vi "Configuration Utility.vi"() -> ()   [LabVIEW 2013, in "RT Temperature Controller.lvlib"]
doc: "This is the main VI for the configuration editor."
uses:
  RT Temperature Controller.lvlib
  Controls/StateCluster.ctl
  <vilib>/NI/Tag Bus Data Framework/Configuration Editor/Classes/SystemConfigRepo/SystemConfigRepo.lvclass
  <vilib>/CEF_TreeControl/Node/NodeRef.ctl
  <vilib>/CEF_TreeControl/Node/NISE_CEF_Node.lvclass
  <vilib>/CEF_TreeControl/Node/UserEventRef.ctl
  <vilib>/CEF_TreeControl/Controls/EventCluster.ctl
  subVI/SplashScreen/splash screen.ctl
  subVI/SplashScreen/notifier data.ctl
  Controls/add message.ctl
  Controls/MoveMessage.ctl
  <vilib>/NI/Tag Bus Module Framework/plugin discovery singleton/class discovery singleton methods.ctl
  <vilib>/NI/Tag Bus Data Framework/Configuration Editor/Classes/Systems/Systems.lvclass
  <vilib>/NI/Tag Bus Data Framework/Framework Configuration Classes/platypus configuration/systems cluster.ctl
  <vilib>/NI/Tag Bus Data Framework/Framework Configuration Classes/system configuration/PL_System Configuration.lvclass
  <vilib>/NI/Tag Bus Data Framework/Framework Configuration Classes/platypus configuration/targets cluster.ctl
  <vilib>/NI/Tag Bus Data Framework/Framework Configuration Classes/target configuration/PL_Target Configuration.lvclass
  <vilib>/NI/Tag Bus Data Framework/Framework Configuration Classes/platypus configuration/engines cluster.ctl
  <vilib>/NI/Module Execution Interface/Engine Configuration/engine configuration.lvclass
  <vilib>/NI/Tag Bus Module Framework/module configuration/TBM module configuration.lvclass
  <vilib>/NI/Tag Bus Data Framework/Configuration Editor/Classes/SystemConfigRepo/SystemConfigRepo.lvclass/SystemConfigRepo.ctl
  <vilib>/CEF_TreeControl/Repository/NISE_CEF_Repository.lvclass
  <vilib>/NI/AMC/Create Single Message.vi
  <vilib>/NI/AMC/Update Message Routing Info.vi
  <vilib>/NI/AMC/Read Termination Message.vi
  <vilib>/NI/Tag Bus Data Framework/Configuration Editor/subVIs/Glyphs Status.ctl
  <vilib>/NI/Tag Bus Data Framework/Configuration Editor/subVIs/Add status to name.vi
  <vilib>/NI/AMC/Send Message.vi
  <vilib>/NI/AMC/Globals.vi
  <vilib>/NI/Tag Bus Data Framework/Configuration Editor/Classes/Module editor node/module editor node.lvclass
  <vilib>/NI/Tag Bus Data Framework/Configuration Editor/Classes/EngineTags/EngineTags.lvclass
  <vilib>/NI/Module Timing Source/timing source/TBM timing source.lvclass
  <vilib>/NI/Tag Bus Data Framework/Configuration Editor/Classes/TBM Configuration Node/TBM Configuration Node.lvclass
  <vilib>/NI/Tag Bus Module Framework/root configuration/TBM configuration.lvclass
  <vilib>/NI/Tag Bus Data Framework/Configuration Editor/Classes/Targets/Targets.lvclass
  <vilib>/NI/Tag Bus Data Framework/Configuration Editor/Classes/Engine Parent/Engine Parent Editor Node.lvclass
  <vilib>/NI/Tag Bus Module Framework/channel/TBM channel.lvclass
  <vilib>/NI/AMC/AMC.lvlib
  <vilib>/CEF_TreeControl/NISE_CEF_TreeControl.lvlib
  subVI/SplashScreen/splash screen.lvlib
  <vilib>/NI/Tag Bus Data Framework/Framework Configuration Classes/class cache/PL_class cache.lvlib
  <vilib>/NI/Tag Bus Module Framework/plugin discovery singleton/class discovery singleton.lvlib
  <vilib>/NI/Tag Bus Data Framework/Configuration Editor/PL Framework Configuration Tool.lvlib
  <vilib>/NI/Tag Bus Data Framework/Framework Configuration Classes/platypus configuration/PLConfigurationSerializer.lvlib
panel:
  in  "Exit":bool
  in  "View":string(tree)
  # "Tag Bus Configuration Editor"
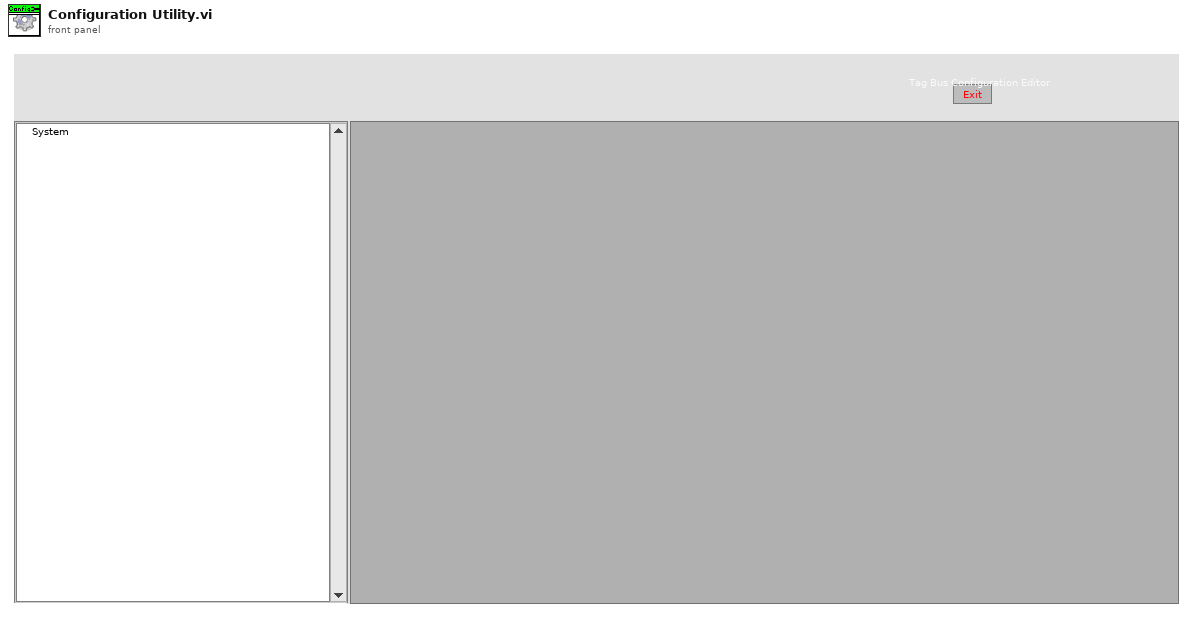
[diagram p1: front panel]
types:
  T1 = enum32{"Invalid", "Standard", "Closed", "Hidden", "Minimized", "Maximized"}
  T2 = typedef "RT Temperature Controller.lvlib/StateCluster.ctl" = cluster{"repository":refnum<class "SystemConfigRepo.lvclass">, "root":T3, "unsaved changes":bool, "current path":path, "user event ref":T4, "glyph path":path[], "SplashScreen":T5, "classes cache":path}
  T3 = typedef "NISE_CEF_Node.lvclass/NodeRef.ctl" = refnum<data-value>
  T4 = typedef "NISE_CEF_Node.lvclass/UserEventRef.ctl" = refnum<user-event>
  T5 = typedef "RT Temperature Controller.lvlib/splash screen.lvlib/splash screen.ctl" = cluster{"reference":refnum<vi>, "update notifier":refnum<notifier>, "Initialized":bool}
  T6 = typedef "AMC.lvlib/Message Queue.ctl" = refnum<queue>
  T7 = typedef "RT Temperature Controller.lvlib/splash screen.lvlib/notifier data.ctl" = cluster{"Text":string, "percent":dbl}
  T8 = typedef "NISE_CEF_TreeControl.lvlib/EventCluster.ctl" = cluster{"command":string, "data":string}
  T9 = typedef "class discovery singleton.lvlib/class discovery singleton methods.ctl" = enum16{"add search paths", "load class by name", "list available classes", "get class path"}
  T10 = typedef "PLConfigurationSerializer.lvlib/systems cluster.ctl" = cluster{"System Configuration":refnum<class "PL_System Configuration.lvclass">, "targets":T11[]}
  T11 = typedef "PLConfigurationSerializer.lvlib/targets cluster.ctl" = cluster{"Target Configuration":refnum<class "PL_Target Configuration.lvclass">, "engines":T12[]}
  T12 = typedef "PLConfigurationSerializer.lvlib/engines cluster.ctl" = cluster{"engine configuration":refnum<class "engine configuration.lvclass">, "modules":refnum<class "TBM module configuration.lvclass">[]}
  T13 = cluster{"node id":string, "RightClickPath":string}
  T14 = typedef "RT Temperature Controller.lvlib/add message.ctl" = cluster{"node type":string, "to add to":string}
  T15 = typedef "RT Temperature Controller.lvlib/MoveMessage.ctl" = cluster{"node ref":T3, "new parent":T3}
  T16 = typedef "RT Temperature Controller.lvlib/FilePaths.ctl" = cluster{"glyphs":path[], "classes":path, "classes cache":path}
  T17 = typedef "PL_class cache.lvlib/cache definition.ctl" = cluster{"configuration":T18, "class cache data":T19}
  T18 = typedef "PL_class cache.lvlib/cache search configuration.ctl" = cluster{"Search Paths":path[], "Folders to Exclude":string[], "full class list":path[]}
  T19 = typedef "PL_class cache.lvlib/cached class information.ctl" = cluster{"targets":T20[], "engines":T21[], "modules":T21[], "ignored class list":path[]}
  T20 = typedef "PL_class cache.lvlib/target class metadata.ctl" = cluster{"file name":string, "fully qualified name":string, "menu display name":string, "configuration class name":string}
  T21 = typedef "PL_class cache.lvlib/class metadata.ctl" = cluster{"file name":string, "fully qualified name":string, "menu display name":string, "configuration class":string, "instances allowed":i32, "supported targets":T22[]}
  T22 = typedef "TBM configuration.lvclass/Target Types.ctl" = enum16{"Windows", "Mac", "Linux", "Linux RT ARM", "VxWorks", "Pharlap", "Other", "Linux RT x64"}
  T23 = typedef "NISE_CEF_Node.lvclass/Summary.ctl" = cluster{"ID":string, "parent ID":string, "node type":string, "text":string, "additional text":string, "glyph":string, "depth":i32}
  T24 = typedef "LVPoint32TypeDef.ctl" = cluster{"Horizontal":i32, "Vertical":i32}
  T25 = cluster{"data name":string, "drag data":variant}[]
  T26 = typedef "NISE_CEF_Node.lvclass/NodeMenuOptions.ctl" = cluster{"removable":bool, "movable":bool, "duplicate":bool}
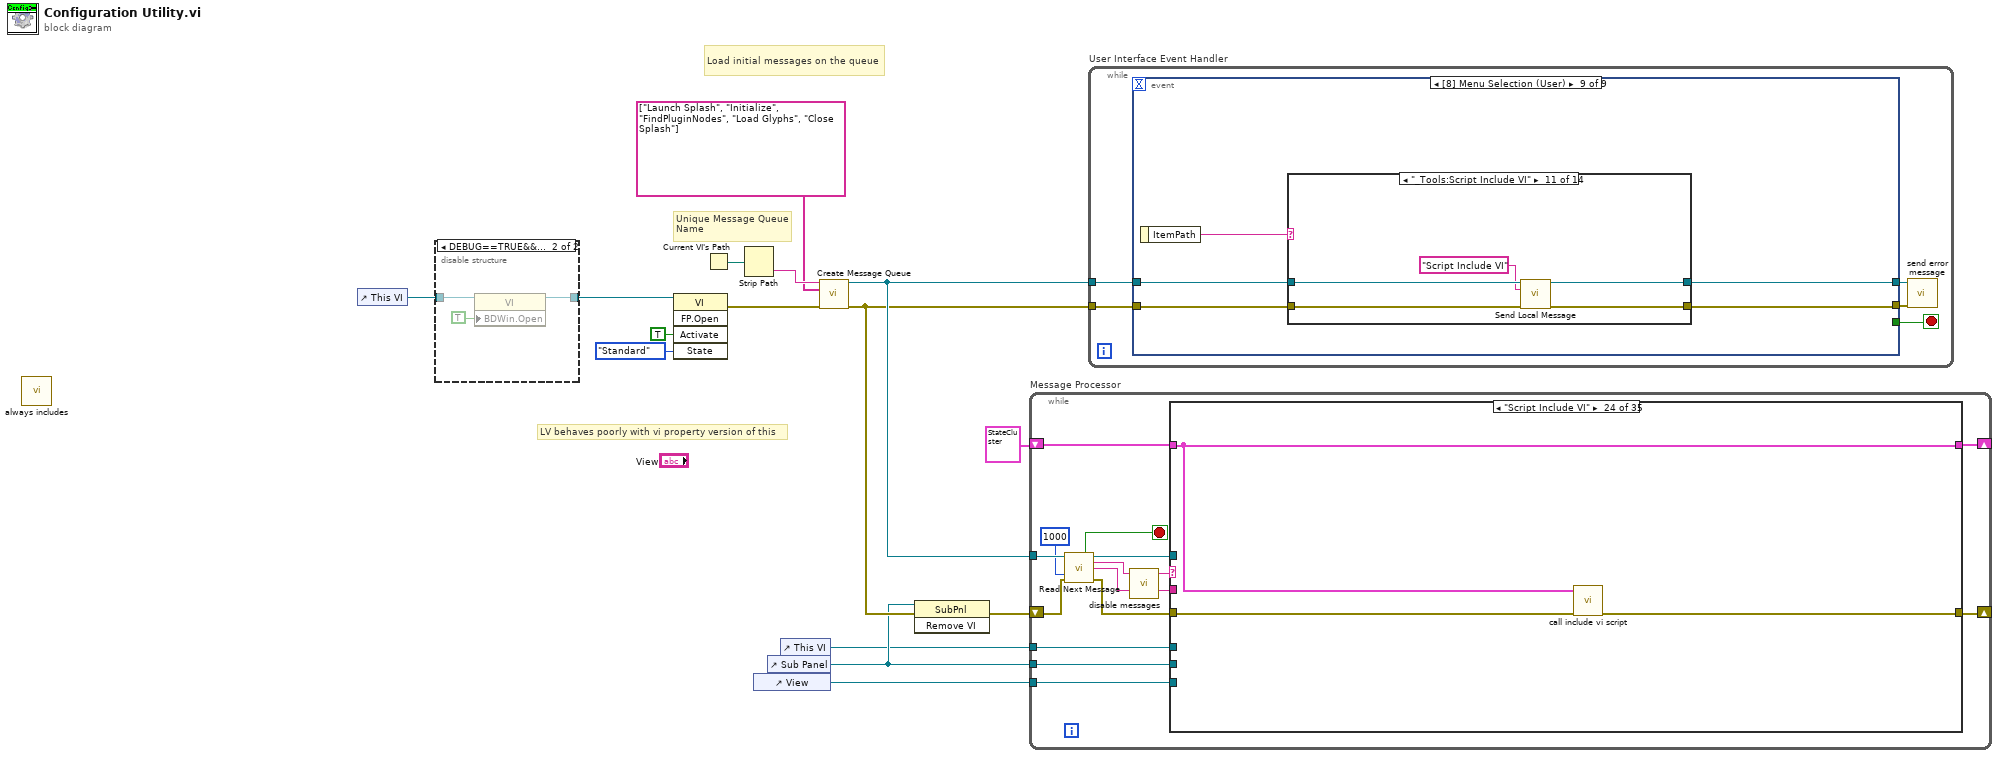
[diagram p0: block diagram]
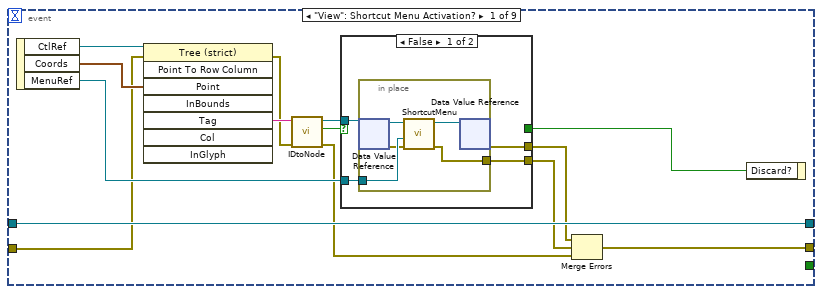
[diagram p3: hidden frame]
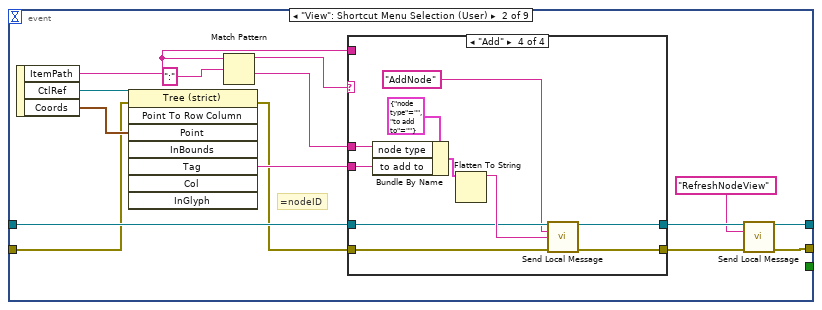
[diagram p5: hidden frame]
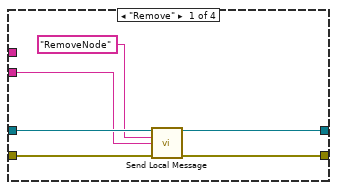
[diagram p6: hidden frame]
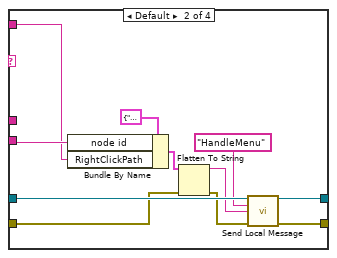
[diagram p7: hidden frame]
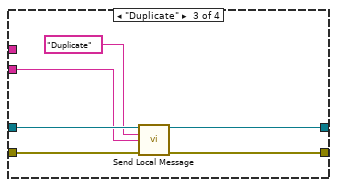
[diagram p8: hidden frame]
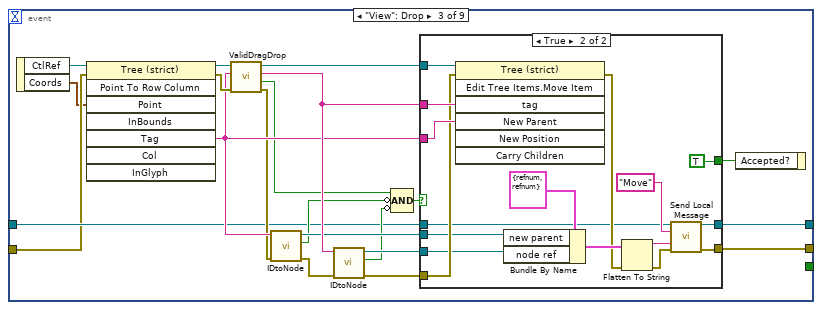
[diagram p9: hidden frame]
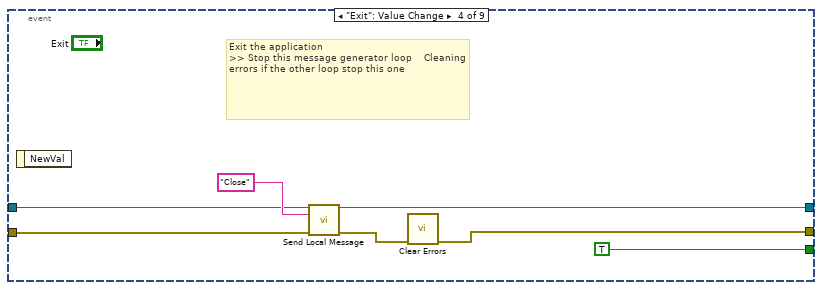
[diagram p11: hidden frame]
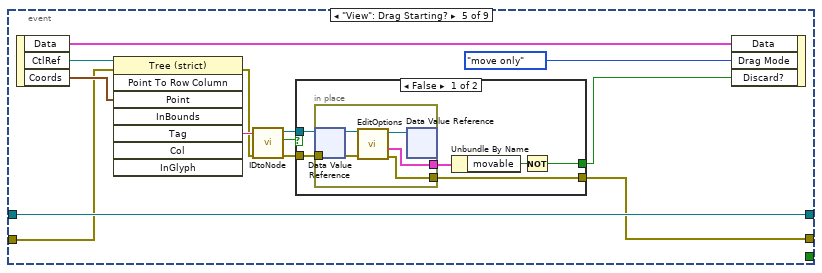
[diagram p12: hidden frame]
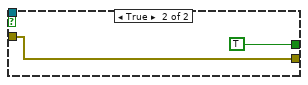
[diagram p13: hidden frame]
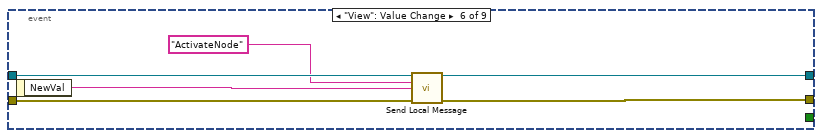
[diagram p14: hidden frame]
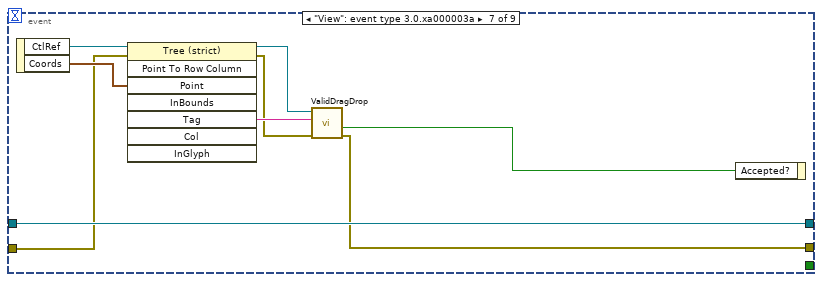
[diagram p15: hidden frame]
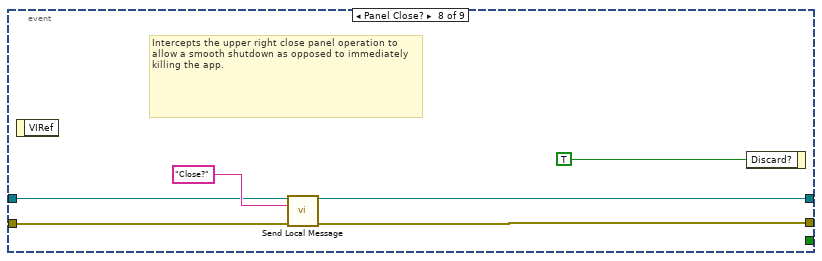
[diagram p16: hidden frame]
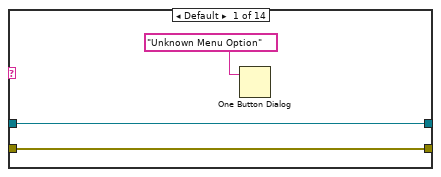
[diagram p17: hidden frame]
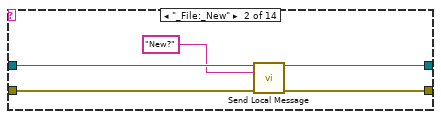
[diagram p18: hidden frame]
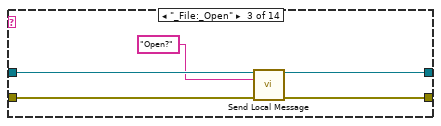
[diagram p19: hidden frame]
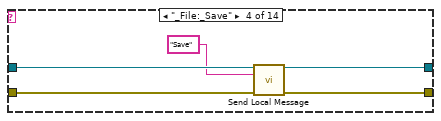
[diagram p20: hidden frame]
diagram:
  # "LV behaves poorly with vi property version of this"
  # "Unique Message Queue Name"
  # "Load initial messages on the queue"
  n1 = call "always includes.vi"() -> ()  [unwired: 12 in]
  n2 = control-ref of="This VI"() -> (w5:refnum<vi>)
  n3 = disable-structure shown="DEBUG==TRUE&&RUN_TIME_ENGINE==False" {
    disable-tunnel: [w16 w19] -> w6
    disable-tunnel: w5 -> [w16 w18]
    frame condition #0 (active) {
    }
    frame condition #1 {
      n4 = property class="VI"(reference=w18, "BDWin.Open"=TRUE ("Block Diagram Window:Open")) -> (reference out=w19:refnum<vi>)  [unwired: 1 in, 1 out]
    }
  }
  n5 = invoke class="VI" method="FP.Open"(reference=w6, "Activate"=TRUE ("Activate?"), "State"=T1."Standard") -> (error out=w9:errorcluster)  [unwired: 2 in, 4 out]
  n6 = Current VI's Path() -> (path=w14:path)
  n7 = Strip Path(path=w14) -> (name=w15:string)  [unwired: 1 out]
  n8 = control-ref of="View"() -> (w4:refnum<vi>)
  n9 = control-ref of="Sub Panel"() -> (w2:refnum<vi>)
  n10 = control-ref of="This VI"() -> (w1:refnum<vi>)
  n11 = call <vilib>:"Create Message Queue.vi"("message queue name"=w15, "initial message names"=string[] ["Launch Splash", "Initialize", "FindPluginNodes", "Load Glyphs", "Close Splash"], "error in"=w9) -> ("message queue out"=w12:T6, "error out"=w10:errorcluster)  [unwired: 11 in]
  n12 = invoke class="SubPnl" method="Remove VI"(reference=w2, error in=w10) -> (error out=w3:errorcluster)  [unwired: 1 in, 2 out]
  n13 = while "Message Processor" {
    shift-right: [w32] -> _
    shift-left: w3 -> [w31]
    tunnel: w12 -> [w30]
    shift-right: [w28] -> _
    shift-left: T2 {"repository"=refnum, "root"=refnum, "unsaved changes"=FALSE, "current path"=path "", "user event ref"=refnum, "glyph path"=[], "SplashScreen"={"reference"=refnum, "update notifier"=refnum, "Initialized"=FALSE}, "classes cache"=path ""} -> [w27]
    tunnel: w1 -> [w22]
    tunnel: w2 -> [w21]
    tunnel: w4 -> [w20]
    stop <- w34 stop-if-true
    n14 = call <vilib>:"Read Next Message.vi"("message queue in"=w30, "timeout (1 ms)"=1000, "error in"=w31) -> ("exit process?"=w34:bool, "message queue out"=w26:T6, "message name"=w23:string, "message value"=w25:string, "error out"=w33:errorcluster)  [unwired: 5 in, 3 out]
    n15 = call "disable messages.vi"("message to check"=w23) -> ("message out"=w24:string)  [unwired: 10 in]
    n16 = case shown="\"Script Include VI\"" w24 {
      selector: w24 -> [_ w38 _ _ _ _ _ _ _ _ _ w156 _ _ _ w278 _ _ _ _ _ _ _ _ _ _ _ _ _ _ _ _ _ _ _]
      tunnel: w25 -> [_ _ _ _ _ _ _ _ w112 _ _ _ _ _ _ _ _ w321 _ _ w383 _ w420 _ _ w461 w473 w491 _ w516 _ _ w563 w586 _]
      tunnel: w33 -> [w36 w41 w43 w50 w69 w76 w97 w103 w113 w139 w143 w153 w190 w202 w237 w270 w297 w326 w343 w348 w381 w395 w422 w437 w440 w459 w472 w492 w504 w515 w541 w551 w562 w585 w591]
      tunnel: [w36 w41 w43 w53 w54 w83 w98 w106 errorcluster {"status"=FALSE, "code"=0, "source"=""} ("error out") w137 w143 w158 w193 w195 w230 w281 w308 w325 w342 w350 w368 w394 w413 w436 w440 w460 w474 w495 w504 w514 w537 w548 w561 w584 w590] -> w32
      tunnel: [w35 w37 w42 w51 w56 w79 w88 w104 w114 w136 w142 w154 w191 w194 w229 w282 w309 w322 w344 w349 w384 w391 w421 w438 w439 w442 w475 w493 w505 w508 w546 w550 w559 w587 w589] -> w28
      tunnel: w27 -> [w35 w37 w42 w52 w70 w79 w89 w104 w114 w136 w142 w155 w189 w203 w238 w277 w304 w323 w344 w349 w384 w392 w421 w438 w439 w458 w475 w494 w506 w508 w546 w550 w559 w587 w589]
      tunnel: w26 -> [_ _ _ _ _ _ w99 w105 w116 w138 _ w157 w192 w201 w236 w267 w307 w324 _ w351 _ w393 w409 _ _ _ _ _ _ _ _ _ w560 w583 _]
      tunnel: w22 -> [_ _ _ w44 w62 _ w86 _ _ _ _ _ _ _ _ _ _ _ _ _ _ _ _ _ _ _ _ _ _ _ w536 _ _ _ _]
      tunnel: w21 -> [_ _ _ _ _ _ _ _ w107 w129 _ w145 _ _ _ w268 w295 _ _ _ _ _ _ _ _ _ _ _ _ w509 _ w547 w552 _ _]
      tunnel: w20 -> [_ _ _ _ _ w82 _ _ _ _ _ w144 _ _ _ _ _ _ _ _ _ _ w408 _ _ w443 w468 w486 _ w510 w540 _ _ _ _]
      frame "", "Idle" {
      }
      frame "Missing Message Handler", Default {
        # "Call this case if a message is received that is not handled by any other case. Typically this is a programming error as a result of a typo or unhandled message/missing message handler."
        n17 = Format Into String(format string="Internal Error: Missing message handler for '%s\" message." ("message"), w38) -> (resulting string=w40:string)  [unwired: 2 in, 1 out]
        n18 = One Button Dialog(message=w40) -> ()  [unwired: 2 out]
      }
      frame "------------Generic Operations------------" {
        # "Dummy case to add a seperation in the Case Structure menu"
      }
      frame "Launch Splash" {
        n19 = invoke class="VI" method="FP.Center"(reference=w44, error in=w50) -> (reference out=w48:refnum<vi>, error out=w47:errorcluster)  [unwired: 1 in, 1 out]
        n20 = invoke class="VI" method="FP.Open"(reference=w48, error in=w47, "State"=T1."Hidden") -> (error out=w45:errorcluster)  [unwired: 2 in, 4 out]
        n21 = call "Launch.vi"("error in"=w45) -> ("error out"=w53:errorcluster, "SplashScreen"=w49:T5)  [unwired: 9 in]
        n22 = Bundle By Name(cluster=w52, "SplashScreen"=w49) -> (w51:T2)
      }
      frame "Initialize" {
        # "issues in exe"
        n23 = Current VI's Menubar() -> (w68:refnum<k9>)
        n24 = call "menu options.vi"("error in"=w69, "VI ref"=w62, "menu ref in"=w68) -> ("error out"=w65:errorcluster)  [unwired: 7 in, 1 out]
        n25 = Create User Event(user event datatype=T8 {"command"="", "data"=""} ("Event"), error in=w65) -> (user event=w66:refnum<user-event>, error out=w54:errorcluster)
        n26 = call "default file paths.vi"() -> ("paths"=w67:T16)  [unwired: 11 in]
        n27 = Unbundle By Name(w67) -> ("classes cache"=w61:path, "glyphs"=w63:path[])
        n28 = Type Cast(type=T4 refnum ("user event ref"), x=w66) -> (*(type *) &x=w60:T4)
        n29 = Bundle By Name(cluster=w70, "user event ref"=w60, "classes cache"=w61, "glyph path"=w63) -> (w56:T2)
        n30 = Unbundle By Name(w56) -> ("SplashScreen"=w55:T5)
        n31 = call "Update.vi"("Update"=T7 {"Text"="Preparing UI...", "percent"=27.0}, "SplashScreen in"=w55) -> ("error out"=w58:errorcluster)  [unwired: 8 in, 1 out]
        n32 = call <vilib>:"Clear Errors.vi"("error in (no error)"=w58) -> ()  [unwired: 6 in, 1 out]
      }
      frame "Load Glyphs" {
        n33 = Unbundle By Name(w79) -> ("SplashScreen"=w78:T5, "glyph path"=w73:path[])
        n34 = call <vilib>:"class discovery singleton.vi"("error in"=w76, "method"=class_discovery_singleton_methods."list available classes") -> ("error out"=w72:errorcluster, "discovered classes"=w75:path[])  [unwired: 6 in, 2 out]
        n35 = for {
          tunnel: w75 -> [w85] mode=indexing
          tunnel: [w84] -> w74 mode=indexing
          n36 = Strip Path(path=w85) -> (stripped path=w84:path)  [unwired: 1 out]
        }
        n37 = Build Array (concatenate)(w73, w74) -> (w71:path[])
        n38 = call "Update.vi"("Update"=T7 {"Text"="Loading Glyphs...", "percent"=78.0}, "SplashScreen in"=w78) -> ("error out"=w81:errorcluster)  [unwired: 8 in, 1 out]
        n39 = call <vilib>:"Clear Errors.vi"("error in (no error)"=w81) -> ()  [unwired: 6 in, 1 out]
        n40 = call "Load Custom Status Glyph.vi"("tree ref"=w82, "error in"=w72, "glyph directories"=w71) -> ("error out"=w83:errorcluster)  [unwired: 8 in]
      }
      frame "Close Splash" {
        n41 = Unbundle By Name(w89) -> ("SplashScreen"=w95:T5)
        n42 = call "Close.vi"("error in"=w97, "SplashScreen"=w95) -> ("error out"=w91:errorcluster, "SplashScreen out"=w87:T5)  [unwired: 8 in]
        n43 = Bundle By Name(cluster=w89, "SplashScreen"=w87) -> (w88:T2)
        n44 = invoke class="VI" method="FP.Open"(reference=w86, error in=w91, "State"=T1."Standard") -> (reference out=w93:refnum<vi>, error out=w92:errorcluster)  [unwired: 2 in, 3 out]
        n45 = Close Reference(reference=w93, error in (no error)=w92) -> (error out=w90:errorcluster)
        n46 = call <vilib>:"Send Local Message.vi"("message queue in"=w99, "message name"="New" ("Message Name"), "error in"=w90) -> ("error out"=w98:errorcluster)  [unwired: 10 in, 2 out]
      }
      frame "Close" {
        n47 = Unbundle By Name(w104) -> ("root"=w101:T3)
        n48 = call <vilib>:"CloseNode.vi"("error in"=w103, "node ref"=w101) -> ("error out"=w100:errorcluster)  [unwired: 9 in]
        n49 = call <vilib>:"Send Local Message.vi"("message queue in"=w105, "message name"="Exit", "error in"=w100) -> ("error out"=w106:errorcluster)  [unwired: 10 in, 2 out]
      }
      frame "Error" {
        n50 = Unbundle By Name(w114) -> ("user event ref"=w110:T4)
        n51 = call "Remove UI without races.vi"("error in"=w113, "user event ref"=w110, "sub panel ref in"=w107) -> ("error out"=w108:errorcluster)  [unwired: 7 in, 1 out]
        n52 = case shown="\"\"" w112 {
          selector: w112 -> [w118 _]
          tunnel: w113 -> [w119 w120]
          tunnel: [w117 w120] -> w109
          frame Default {
            n53 = Unflatten From String(type=w119, binary string=w118, error in (no error)=w119) -> (value=w117:errorcluster)  [unwired: 2 in, 2 out]
          }
          frame "" {
          }
        }
        n54 = call <vilib>:"Clear Errors.vi"("error in (no error)"=w108) -> ()  [unwired: 6 in, 1 out]
        n55 = Unbundle By Name(w109) -> ("code"=w111:i32)
        n56 = case shown="15550" w111 {
          tunnel: w116 -> [_ _ _ w126 _]
          tunnel: w109 -> [_ _ _ w125 w128]
          frame -2147220623, -2147220621, -2147220364, 56, 63 {
            n57 = One Button Dialog(message="Problem communicating with remote device.  Make sure a valid device is selected and that the IP address is correct.") -> ()  [unwired: 1 in, 1 out]
          }
          frame 1003 {
            n58 = One Button Dialog(message="Dev Error: The Ui.vi for the selected class is broken") -> ()  [unwired: 1 in, 1 out]
          }
          frame 15550 {
            n59 = One Button Dialog(message="The cRIO does not yet have a configuration to download. Create or open a configuration and download it to the cRIO") -> ()  [unwired: 1 in, 1 out]
          }
          frame 537549 {
            n60 = call <vilib>:"Send Local Message.vi"("message queue in"=w126, "message name"="Exit", "error in"=w125) -> ()  [unwired: 10 in, 3 out]
            n61 = One Button Dialog(message="Invalid configuration file.") -> ()  [unwired: 1 in, 1 out]
          }
          frame 1, Default {
            n62 = call <vilib>:"Simple Error Handler.vi"("error in (no error)"=w128) -> ()  [unwired: 1 in, 8 out]
          }
        }
      }
      frame "Exit" {
        # "Stop the VI                                                                             >> Perform any cleanup tasks in this message case. >> Clear display before closing."
        n63 = call <vilib>:"Destroy Message Queue.vi"("message queue in"=w138, "error in"=w139) -> ("error out"=w133:errorcluster)  [unwired: 11 in, 2 out]
        n64 = control-ref of="Exit"() -> (w135:refnum<vi>)
        n65 = Unbundle By Name(w136) -> ("user event ref"=w130:T4)
        n66 = property class="Bool (strict)"(reference=w135, error in=w133, "Val(Sgnl)"=FALSE ("Exit")) -> (error out=w132:errorcluster)  [unwired: 1 out]
        n67 = call "Remove UI without races.vi"("error in"=w132, "user event ref"=w130, "sub panel ref in"=w129) -> ("error out"=w131:errorcluster)  [unwired: 7 in, 1 out]
        n68 = disable-structure shown="RUN_TIME_ENGINE==True" {
          disable-tunnel: [w140 w141] -> w137
          disable-tunnel: w131 -> [w140 w141]
          frame condition #0 (active) {
          }
          frame condition #1 {
            n69 = Quit LabVIEW() -> ()  [unwired: 1 in]
          }
        }
      }
      frame "------------Menu Operations--------------" {
        # "Dummy case to add a seperation in the Case Structure menu"
      }
      frame "Close?", "New?", "Open?" {
        n70 = Unbundle By Name(w155) -> ("unsaved changes"=w146:bool, "user event ref"=w147:T4)
        n71 = case shown="True" w146 {
          tunnel: [TRUE ("SaveFlag") w176] -> w149
          tunnel: w155 -> [w168 w175]
          tunnel: [w168 w174] -> w154
          tunnel: w153 -> [w167 w173]
          tunnel: [w167 w172] -> w148
          tunnel: w145 -> [_ w171]
          tunnel: w144 -> [_ w170]
          frame False {
            # "If there is nothing to save Go do Action"
          }
          frame True {
            n72 = call "dialog save dirty dot.vi"("error in"=w173, "View"=w170, "sub panel ref in"=w171, "state in"=w175) -> ("error out"=w172:errorcluster, "new"=w176:bool, "state out"=w174:T2)  [unwired: 5 in]
          }
        }
        n73 = Search and Replace String(input string=w156, search string="?", replace string="") -> (result string=w150:string)  [unwired: 5 in, 3 out]
        n74 = case shown="True" w149 {
          tunnel: w148 -> [w159 w166]
          tunnel: [w159 w162] -> w158
          tunnel: w157 -> [_ w165]
          tunnel: w150 -> [_ w164]
          tunnel: w147 -> [_ w161]
          tunnel: w145 -> [_ w160]
          frame False {
          }
          frame True {
            n75 = call <vilib>:"Send Local Message.vi"("message queue in"=w165, "message name"=w164, "error in"=w166) -> ("error out"=w163:errorcluster)  [unwired: 10 in, 2 out]
            n76 = call "Remove UI without races.vi"("error in"=w163, "user event ref"=w161, "sub panel ref in"=w160) -> ("error out"=w162:errorcluster)  [unwired: 7 in, 1 out]
          }
        }
      }
      frame "New" {
        # "unused"
        n77 = call <vilib>:"create default cache.vi"() -> ("cache"=w179:T17)  [unwired: 11 in]
        n78 = Unbundle By Name(w179) -> ("configuration.Search Paths"=w178:path[])
        n79 = call-dynamic "Initialize.vi"("error in"=w190, "node in"=refnum<class "Systems.lvclass"> refnum ("Systems.lvclass")) -> ("error out"=w185:errorcluster, "data value reference"=w186:T3)  [unwired: 7 in, 1 out]
        n80 = Delete From Array(array=w178) -> (deleted portion=w177:path)  [unwired: 2 in, 1 out]
        n81 = call-dynamic "Initialize.vi"("error in"=w185, "path"=w177, "repository in"=refnum<class "SystemConfigRepo.lvclass"> refnum ("SystemConfigRepo.lvclass")) -> ("error out"=w184:errorcluster, "repository out"=w183:refnum<class "SystemConfigRepo.lvclass">)  [unwired: 7 in]
        n82 = Bundle By Name(cluster=w189, "unsaved changes"=FALSE ("SaveFlag"), "repository"=w183, "root"=w186, "current path"=path "") -> (w191:T2)
        n83 = call <vilib>:"Send Local Message.vi"("message queue in"=w192, "message name"="PopulateTree", "error in"=w184) -> ("error out"=w193:errorcluster)  [unwired: 10 in, 2 out]
      }
      frame "Open" {
        n84 = call <vilib>:"Set Busy.vi"() -> ("error out"=w198:errorcluster)  [unwired: 10 in, 1 out]
        n85 = call "File Dialog"("pattern (all files)"="*.pcfg") -> ("selected path"=w200:path, "cancelled"=w199:bool)  [unwired: 11 in, 2 out]
        n86 = case shown="False" w199 {
          tunnel: w203 -> [w212 w228]
          tunnel: [w211 w228] -> w194
          tunnel: w202 -> [w210 w227]
          tunnel: w201 -> [w209 _]
          tunnel: [w208 w227] -> w195
          tunnel: w200 -> [w205 _]
          tunnel: w198 -> [w204 w226]
          tunnel: [w204 w226] -> w197
          frame False {
            n87 = in-place {
              in-place-border: w210 -> [w225]
              in-place-border: [w214] -> w206
              in-place-border: w205 -> [w220]
              n88 = in-place-cluster #1(w212) -> ("repository"=w213:refnum<class "SystemConfigRepo.lvclass">, "current path"=w221:path)  [unwired: 2 out]
              n89 = call-dynamic "Open.vi"("error in"=w225, "file path"=w220, "SystemConfigRepo in"=w213) -> ("error out"=w222:errorcluster, "SystemConfigRepo out"=w218:refnum<class "SystemConfigRepo.lvclass">)  [unwired: 6 in, 1 out]
              n90 = call-dynamic "WriteTree.vi"("error in"=w222, "SystemConfigRepo in"=w218) -> ("error out"=w215:errorcluster, "root"=w223:T3, "repository out"=w217:refnum<class "NISE_CEF_Repository.lvclass">)  [unwired: 7 in]
              n91 = To More Specific Class(target class=w213, reference=w217, error in=w215) -> (specific class reference=w216:refnum<class "SystemConfigRepo.lvclass">, error out=w214:errorcluster)
              n92 = Select(t=w221, s=w214, f=w220) -> (s? t:f=w219:path)
              n93 = in-place-cluster #1("unsaved changes"=FALSE ("SaveFlag"), "repository"=w216, "root"=w223, "current path"=w219) -> (w211:T2)
            }
            n94 = call <vilib>:"Send Local Message.vi"("message queue in"=w209, "message name"="PopulateTree", "error in"=w206) -> ("error out"=w208:errorcluster)  [unwired: 10 in, 2 out]
          }
          frame True {
          }
        }
        n95 = call <vilib>:"Unset Busy.vi"("error in (no error)"=w197) -> ()  [unwired: 10 in, 1 out]
      }
      frame "Load Binary" {
        n96 = call <vilib>:"Set Busy.vi"() -> ("error out"=w233:errorcluster)  [unwired: 10 in, 1 out]
        n97 = call "File Dialog2"("pattern (all files)"="*.pbin") -> ("selected path"=w235:path, "cancelled"=w234:bool)  [unwired: 11 in, 2 out]
        n98 = case shown="False" w234 {
          tunnel: w238 -> [w247 w266]
          tunnel: [w246 w266] -> w229
          tunnel: w237 -> [w245 w265]
          tunnel: w236 -> [w244 _]
          tunnel: [w243 w265] -> w230
          tunnel: w235 -> [w240 _]
          tunnel: w233 -> [w239 w264]
          tunnel: [w239 w264] -> w232
          frame False {
            n99 = in-place {
              in-place-border: w245 -> [w254]
              in-place-border: [w258] -> w241
              in-place-border: w240 -> [w250]
              n100 = in-place-cluster #2(w247) -> ("repository"=w256:refnum<class "SystemConfigRepo.lvclass">)  [unwired: 2 out]
              n101 = Read from Binary File(5:T10 {"System Configuration"=refnum, "targets"=[]} ("system"), 8:w254, 11:w250) -> (0:w253:errorcluster, 2:w251:T10, 3:w248:refnum<file>)  [unwired: 3 in, 1 out]
              n102 = Close File(refnum=w248, error in=w253) -> (error out=w249:errorcluster)  [unwired: 1 out]
              n103 = call <vilib>:"Write Systems.vi"("error in"=w249, "system"=w251, "SystemConfigRepo in"=w256) -> ("error out"=w255:errorcluster, "SystemConfigRepo out"=w257:refnum<class "SystemConfigRepo.lvclass">)  [unwired: 7 in]
              n104 = call-dynamic "WriteTree.vi"("error in"=w255, "SystemConfigRepo in"=w257) -> ("error out"=w259:errorcluster, "root"=w262:T3, "repository out"=w261:refnum<class "NISE_CEF_Repository.lvclass">)  [unwired: 7 in]
              n105 = To More Specific Class(target class=w256, reference=w261, error in=w259) -> (specific class reference=w260:refnum<class "SystemConfigRepo.lvclass">, error out=w258:errorcluster)
              n106 = in-place-cluster #2("unsaved changes"=TRUE ("SaveFlag"), "repository"=w260, "root"=w262) -> (w246:T2)
            }
            n107 = call <vilib>:"Send Local Message.vi"("message queue in"=w244, "message name"="PopulateTree", "error in"=w241) -> ("error out"=w243:errorcluster)  [unwired: 10 in, 2 out]
          }
          frame True {
          }
        }
        n108 = call <vilib>:"Unset Busy.vi"("error in (no error)"=w232) -> ()  [unwired: 10 in, 1 out]
      }
      frame "Save", "SaveAs" {
        n109 = Unbundle By Name(w277) -> ("user event ref"=w271:T4)
        n110 = call <vilib>:"Set Busy.vi"() -> ("error out"=w275:errorcluster)  [unwired: 10 in, 1 out]
        n111 = call "Remove UI without races.vi"("error in"=w270, "user event ref"=w271, "sub panel ref in"=w268) -> ("error out"=w269:errorcluster)  [unwired: 7 in, 1 out]
        n112 = flat-sequence {
          tunnel: w269 -> [w289]
          tunnel: w278 -> [w287]
          tunnel: w277 -> [w284]
          tunnel: w275 -> [w283]
          tunnel: [w290] -> w274
          tunnel: [w288] -> w273
          tunnel: [w283] -> w272
          tunnel: [w292] -> w276
          tunnel: [w293] -> w279
          tunnel: [w294] -> w282
          tunnel: w274 -> [w294]
          tunnel: w273 -> [w293]
          tunnel: w272 -> [w292]
          frame #0 {
            n113 = Equal?(x="SaveAs", y=w287) -> (x = y?=w286:bool)
            n114 = call "save operation.vi"("force save as"=w286, "error in"=w289, "state cluster"=w284) -> ("error out"=w288:errorcluster, "state out"=w290:T2)  [unwired: 7 in]
          }
          frame #1 {
            n115 = local read "View"() -> (w291:string)
            n116 = property on="View" class="Tree (strict)"("Val(Sgnl)"=w291) -> ()  [unwired: 2 in, 2 out]
          }
        }
        n117 = call <vilib>:"Unset Busy.vi"("error in (no error)"=w276) -> ()  [unwired: 10 in, 1 out]
        n118 = call <vilib>:"Send Local Message.vi"("message queue in"=w267, "message name"="PopulateTree", "error in"=w279) -> ("error out"=w281:errorcluster)  [unwired: 10 in, 2 out]
      }
      frame "Save Binary" {
        n119 = Unbundle By Name(w304) -> ("user event ref"=w298:T4)
        n120 = call <vilib>:"Set Busy.vi"() -> ("error out"=w302:errorcluster)  [unwired: 10 in, 1 out]
        n121 = call "Remove UI without races.vi"("error in"=w297, "user event ref"=w298, "sub panel ref in"=w295) -> ("error out"=w296:errorcluster)  [unwired: 7 in, 1 out]
        n122 = flat-sequence {
          tunnel: w296 -> [w313]
          tunnel: w304 -> [w310]
          tunnel: w302 -> [w314]
          tunnel: [w311] -> w301
          tunnel: [w312] -> w300
          tunnel: [w314] -> w299
          tunnel: [w316] -> w303
          tunnel: [w317] -> w305
          tunnel: [w318] -> w309
          tunnel: w301 -> [w318]
          tunnel: w300 -> [w317]
          tunnel: w299 -> [w316]
          frame #0 {
            n123 = call "save operation binary.vi"("error in"=w313, "state cluster"=w310) -> ("error out"=w312:errorcluster, "state out"=w311:T2)  [unwired: 8 in]
          }
          frame #1 {
            n124 = local read "View"() -> (w315:string)
            n125 = property on="View" class="Tree (strict)"("Val(Sgnl)"=w315) -> ()  [unwired: 2 in, 2 out]
          }
        }
        n126 = call <vilib>:"Unset Busy.vi"("error in (no error)"=w303) -> ()  [unwired: 10 in, 1 out]
        n127 = call <vilib>:"Send Local Message.vi"("message queue in"=w307, "message name"="PopulateTree", "error in"=w305) -> ("error out"=w308:errorcluster)  [unwired: 10 in, 2 out]
      }
      frame "Custom View" {
        n128 = in-place {
          in-place-border: w326 -> [w339]
          in-place-border: [w330] -> w319
          in-place-border: w321 -> [w331]
          n129 = in-place-cluster #3(w323) -> ("repository"=w328:refnum<class "SystemConfigRepo.lvclass">, "root"=w337:T3)
          n130 = call-dynamic "ReadTree.vi"("error in"=w339, "root"=w337, "SystemConfigRepo in"=w328) -> ("error out"=w335:errorcluster, "repository out"=w333:refnum<class "NISE_CEF_Repository.lvclass">)  [unwired: 7 in]
          n131 = call-dynamic "CustomView.vi"("error in"=w335, "view name"=w331, "repository in"=w333) -> ("error out"=w334:errorcluster, "repository out"=w332:refnum<class "NISE_CEF_Repository.lvclass">)  [unwired: 7 in]
          n132 = call-dynamic "WriteTree.vi"("error in"=w334, "repository in"=w332) -> ("error out"=w338:errorcluster, "root"=w336:T3, "repository out"=w329:refnum<class "NISE_CEF_Repository.lvclass">)  [unwired: 7 in]
          n133 = To More Specific Class(target class=w328, reference=w329, error in=w338) -> (specific class reference=w327:refnum<class "SystemConfigRepo.lvclass">, error out=w330:errorcluster)
          n134 = in-place-cluster #3("repository"=w327, "root"=w336) -> (w322:T2)
        }
        n135 = call <vilib>:"Send Local Message.vi"("message queue in"=w324, "message name"="PopulateTree", "error in"=w319) -> ("error out"=w325:errorcluster)  [unwired: 10 in, 2 out]
      }
      frame "DeployTool" {
        n136 = Unbundle By Name(w344) -> ("current path"=w340:path, "root"=w341:T3)
        n137 = call <vilib>:"deployment tool.vi"("current pcfg path"=w340, "error in"=w343, "node ref"=w341) -> ("error out"=w342:errorcluster)  [unwired: 8 in]
      }
      frame "Edit Plugin Search Paths" {
        n138 = Unbundle By Name(w349) -> ("classes cache"=w345:path)
        n139 = call <vilib>:"load cache.vi"("error in"=w348, "cache path"=w345) -> ("error out"=w346:errorcluster, "cache"=w347:T17)  [unwired: 8 in]
        n140 = Unbundle By Name(w347) -> ("configuration.Search Paths"=w355:path[])
        n141 = call "dialog edit search paths.vi"("error in"=w346, "Plugin Search Paths"=w355) -> ("error out"=w352:errorcluster, "Cancelled?"=w354:bool, "Plugin Search Paths"=w353:path[])  [unwired: 7 in]
        n142 = case shown="False" w354 {
          tunnel: w347 -> [w365 _]
          tunnel: w353 -> [w364 _]
          tunnel: w352 -> [w358 w366]
          tunnel: w351 -> [w361 _]
          tunnel: [w360 w366] -> w350
          tunnel: w345 -> [w356 _]
          frame False {
            n143 = Bundle By Name(cluster=w365, "configuration.Search Paths"=w364) -> (w357:T17)
            n144 = call <vilib>:"save cache.vi"("error in"=w358, "cache"=w357, "path"=w356) -> ("error out"=w359:errorcluster)  [unwired: 8 in]
            n145 = call <vilib>:"Send Local Message.vi"("message queue in"=w361, "message name"="FindPluginNodes", "message value"="Refresh", "error in"=w359) -> ("error out"=w360:errorcluster)  [unwired: 9 in, 2 out]
          }
          frame True {
          }
        }
      }
      frame "FindPluginNodes" {
        n146 = call <vilib>:"Set Busy.vi"("error in (no error)"=w381) -> ("error out"=w380:errorcluster)  [unwired: 9 in, 1 out]
        n147 = Unbundle By Name(w384) -> ("SplashScreen"=w374:T5, "classes cache"=w370:path)
        n148 = Equal?(x="Refresh", y=w383) -> (x = y?=w375:bool)
        n149 = call <vilib>:"load cache.vi"("error in"=w380, "cache path"=w370) -> ("error out"=w379:errorcluster, "cache"=w378:T17)  [unwired: 8 in]
        n150 = case shown="Error" w379 {
          selector: w379 -> [w387 _]
          tunnel: [w385 w388] -> w376
          tunnel: w378 -> [w386 _]
          tunnel: [w387 _] -> w377
          frame No Error {
            n151 = call <vilib>:"remove missing files.vi"("cache in"=w386) -> ("cache out"=w385:T17)  [unwired: 10 in]
          }
          frame Error {
            n152 = call <vilib>:"create default cache.vi"() -> ("cache"=w388:T17)  [unwired: 11 in]
          }
        }
        n153 = call <vilib>:"identify new classes.vi"("error in"=w377, "force scan"=w375, "cache in"=w376) -> ("error out"=w371:errorcluster, "cache out"=w367:T17)  [unwired: 7 in]
        n154 = call "Update.vi"("Update"=T7 {"Text"="Loading Classes...", "percent"=45.0}, "SplashScreen in"=w374) -> ("error out"=w373:errorcluster)  [unwired: 8 in, 1 out]
        n155 = call <vilib>:"Clear Errors.vi"("error in (no error)"=w373) -> ()  [unwired: 6 in, 1 out]
        n156 = call <vilib>:"save cache.vi"("error in"=w371, "cache"=w367, "path"=w370) -> ("error out"=w369:errorcluster)  [unwired: 8 in]
        n157 = call <vilib>:"Unset Busy.vi"("error in (no error)"=w369) -> ("error out"=w368:errorcluster)  [unwired: 10 in]
      }
      frame "Test" {
        n158 = in-place {
          in-place-border: w395 -> [w407]
          in-place-border: [w402] -> w389
          n159 = in-place-cluster #4(w392) -> ("repository"=w397:refnum<class "SystemConfigRepo.lvclass">, "root"=w404:T3)
          n160 = call-dynamic "ReadTree.vi"("error in"=w407, "root"=w404, "SystemConfigRepo in"=w397) -> ("error out"=w403:errorcluster, "repository out"=w399:refnum<class "NISE_CEF_Repository.lvclass">)  [unwired: 7 in]
          n161 = To More Specific Class(target class=w397, reference=w399, error in=w403) -> (specific class reference=w398:refnum<class "SystemConfigRepo.lvclass">, error out=w400:errorcluster)
          n162 = call-dynamic "WriteTree.vi"("error in"=w400, "SystemConfigRepo in"=w398) -> ("error out"=w406:errorcluster, "root"=w405:T3, "repository out"=w401:refnum<class "NISE_CEF_Repository.lvclass">)  [unwired: 7 in]
          n163 = To More Specific Class(target class=w397, reference=w401, error in=w406) -> (specific class reference=w396:refnum<class "SystemConfigRepo.lvclass">, error out=w402:errorcluster)
          n164 = in-place-cluster #4("repository"=w396, "root"=w405) -> (w391:T2)
        }
        n165 = call <vilib>:"Send Local Message.vi"("message queue in"=w393, "message name"="PopulateTree", "error in"=w389) -> ("error out"=w394:errorcluster)  [unwired: 10 in, 2 out]
      }
      frame "HandleMenu" {
        n166 = Unflatten From String(type=T13 {"node id"="", "RightClickPath"=""} ("input cluster"), binary string=w420, error in (no error)=w422) -> (value=w418:T13, error out=w417:errorcluster)  [unwired: 2 in, 1 out]
        n167 = Unbundle By Name(w418) -> ("RightClickPath"=w411:string, "node id"=w416:string)
        n168 = call <vilib>:"IDtoNode.vi"("error in"=w417, "ID"=w416) -> ("error out"=w414:errorcluster, "node ref"=w415:T3)  [unwired: 7 in, 1 out]
        n169 = in-place {
          in-place-border: w414 -> [w435]
          in-place-border: [w430] -> w413
          in-place-border: [w429] -> w412
          in-place-border: w411 -> [w428]
          in-place-border: [w428] -> w410
          in-place-border: w409 -> [w427]
          in-place-border: w408 -> [w426]
          n170 = in-place-dvr #5(w415) -> (w432:refnum<class "NISE_CEF_Node.lvclass">, w434:errorcluster)
          n171 = Merge Errors(w435, w434) -> (w433:errorcluster)
          n172 = call-dynamic "MenuHandler.vi"("tree control"=w426, "message queue out"=w427, "error in (no error)"=w433, "menu string"=w428, "NISE_CEF_Node in"=w432) -> ("error out"=w430:errorcluster, "Unhandled"=w429:bool, "NISE_CEF_Node out"=w431:refnum<class "NISE_CEF_Node.lvclass">)  [unwired: 4 in]
          n173 = in-place-dvr #5(w431) -> ()  [unwired: 2 out]
        }
        n174 = case shown="True" w412 {
          tunnel: w410 -> [_ w423]
          frame False {
          }
          frame True {
            n175 = Concatenate Strings("Unknown item path:\n" ("message"), w423) -> (w425:string)
            n176 = One Button Dialog(message=w425) -> ()  [unwired: 1 in, 1 out]
          }
        }
      }
      frame "Script Include VI" {
        n177 = call "call include vi script.vi"("error in (no error)"=w437, "state cluster"=w438) -> ("error out"=w436:errorcluster)  [unwired: 9 in]
      }
      frame "-------TreeControl Operations-----------" {
        # "Dummy case to add a seperation in the Case Structure menu"
      }
      frame "AddNode" {
        n178 = call <vilib>:"Set Busy.vi"("error in (no error)"=w459) -> ("error out"=w444:errorcluster)  [unwired: 9 in, 1 out]
        n179 = Unflatten From String(type=T14 {"node type"="", "to add to"=""} ("input cluster"), binary string=w461) -> (value=w454:T14)  [unwired: 3 in, 2 out]
        n180 = Unbundle By Name(w454) -> ("to add to"=w451:string, "node type"=w447:string)
        n181 = in-place {
          in-place-border: w447 -> [w467]
          in-place-border: [w464] -> w446
          in-place-border: w444 -> [w463]
          in-place-border: [w462] -> w445
          n182 = in-place-cluster #6(w458) -> ("repository"=w466:refnum<class "SystemConfigRepo.lvclass">)
          n183 = call-dynamic "GetClassPath.vi"("error in"=w463, "class name"=w467, "SystemConfigRepo in"=w466) -> ("error out"=w462:errorcluster, "class path"=w464:path, "SystemConfigRepo out"=w465:refnum<class "SystemConfigRepo.lvclass">)  [unwired: 6 in]
          n184 = in-place-cluster #6("repository"=w465) -> (w442:T2)
        }
        n185 = call <vilib>:"Get LV Class Default Value.vi"("error in (no error)"=w445, "class path"=w446) -> ("error out"=w456:errorcluster, "object"=w457:refnum<class>)  [unwired: 8 in]
        n186 = To More Specific Class(target class=refnum<class "NISE_CEF_Node.lvclass"> refnum ("NISE_CEF_Node.lvclass"), reference=w457, error in=w456) -> (specific class reference=w453:refnum<class "NISE_CEF_Node.lvclass">, error out=w450:errorcluster)
        n187 = call <vilib>:"AddNode.vi"("error in"=w450, "node in"=w453, "parent node ID"=w451) -> ("error out"=w449:errorcluster, "summary"=w448:T23[])  [unwired: 7 in]
        n188 = call <vilib>:"PopulateTreeSumary.vi"("error in"=w449, "array"=w448, "tree ref in"=w443) -> ("error out"=w441:errorcluster)  [unwired: 8 in]
        n189 = call <vilib>:"Unset Busy.vi"("error in (no error)"=w441) -> ("error out"=w460:errorcluster)  [unwired: 10 in]
      }
      frame "Duplicate" {
        n190 = call <vilib>:"IDtoNode.vi"("error in"=w472, "ID"=w473) -> ("error out"=w470:errorcluster, "invalid Id"=w469:bool, "node ref"=w471:T3)  [unwired: 7 in]
        n191 = case shown="False" w469 {
          tunnel: [w484 w485] -> w474
          tunnel: w471 -> [w483 _]
          tunnel: w470 -> [w480 w485]
          tunnel: w468 -> [w476 _]
          frame False {
            n192 = call <vilib>:"DuplicateNode.vi"("same parent?"=TRUE ("s"), "error in"=w480, "node ref in"=w483) -> ("error out"=w481:errorcluster, "new node ref"=w482:T3)  [unwired: 7 in]
            n193 = call <vilib>:"Summary.vi"("error in"=w481, "node self ref"=w482) -> ("error out"=w478:errorcluster, "summary"=w477:T23[])  [unwired: 8 in]
            n194 = call <vilib>:"PopulateTreeSumary.vi"("error in"=w478, "array"=w477, "tree ref in"=w476) -> ("error out"=w484:errorcluster)  [unwired: 8 in]
          }
          frame True {
          }
        }
      }
      frame "RefreshNode" {
        # "Refreshes the node in the Tree               Sets the save flag to true                       This case can be called from the UIs of the nodes"
        n195 = call <vilib>:"IDtoNode.vi"("error in"=w492, "ID"=w491) -> ("error out"=w489:errorcluster, "invalid Id"=w487:bool, "node ref"=w488:T3)  [unwired: 7 in]
        n196 = case shown="False" w487 {
          tunnel: [w501 w502] -> w495
          tunnel: w489 -> [w498 w502]
          tunnel: w488 -> [w497 _]
          tunnel: w486 -> [w496 _]
          frame False {
            n197 = call <vilib>:"Summary.vi"("error in"=w498, "node self ref"=w497) -> ("error out"=w500:errorcluster, "summary"=w499:T23[])  [unwired: 8 in]
            n198 = call <vilib>:"RefreshSubTree.vi"("error in"=w500, "node information"=w499, "tree ref in"=w496) -> ("error out"=w501:errorcluster)  [unwired: 7 in, 1 out]
          }
          frame True {
          }
        }
        n199 = Bundle By Name(cluster=w494, "unsaved changes"=TRUE ("SaveFlag")) -> (w493:T2)
      }
      frame "SetDirtyDot" {
        n200 = Bundle By Name(cluster=w506, "unsaved changes"=TRUE ("SaveFlag")) -> (w505:T2)
      }
      frame "RemoveNode" {
        n201 = Unbundle By Name(w508) -> ("user event ref"=w507:T4)
        n202 = call <vilib>:"IDtoNode.vi"("error in"=w515, "ID"=w516) -> ("error out"=w513:errorcluster, "invalid Id"=w511:bool, "node ref"=w512:T3)  [unwired: 7 in]
        n203 = case shown="True" w511 {
          tunnel: w513 -> [w524 w534]
          tunnel: w512 -> [w522 _]
          tunnel: [w526 w534] -> w514
          tunnel: w510 -> [w525 _]
          tunnel: w509 -> [w521 _]
          tunnel: w507 -> [w520 _]
          frame False {
            n204 = call "check if subpanel should be closed.vi"("error in"=w524, "SubPanel in"=w521, "node in"=w522) -> ("error out"=w519:errorcluster, "needs closing"=w517:bool, "node out"=w523:T3)  [unwired: 6 in]
            n205 = case shown="True" w517 {
              tunnel: w521 -> [_ w533]
              tunnel: w520 -> [_ w532]
              tunnel: w519 -> [w529 w531]
              tunnel: [w529 w530] -> w518
              frame False {
              }
              frame True {
                n206 = call "Remove UI without races.vi"("error in"=w531, "user event ref"=w532, "sub panel ref in"=w533) -> ("error out"=w530:errorcluster)  [unwired: 7 in, 1 out]
              }
            }
            n207 = call <vilib>:"RemoveNode.vi"("error in"=w518, "node"=w523) -> ("error out"=w527:errorcluster, "node ID"=w528:string)  [unwired: 8 in]
            n208 = call <vilib>:"ClearTreeNode.vi"("error in"=w527, "tag"=w528, "tree reference"=w525) -> ("error out"=w526:errorcluster)  [unwired: 8 in]
          }
          frame True {
          }
        }
      }
      frame "PopulateTree" {
        n209 = Unbundle By Name(w546) -> ("current path"=w539:path, "root"=w543:T3)
        n210 = call <vilib>:"Summary.vi"("error in"=w541, "depth"=0 ("Depth"), "node self ref"=w543) -> ("error out"=w544:errorcluster, "summary"=w545:T23[])  [unwired: 7 in]
        n211 = Strip Path(path=w539) -> (name=w535:string)  [unwired: 1 out]
        n212 = call <vilib>:"RefreshEntireTree.vi"("calling VI in"=w536, "error in"=w544, "array"=w545, "tree ref in"=w540) -> ("error out"=w538:errorcluster)  [unwired: 7 in]
        n213 = property class="VI"(reference=w536, error in=w538, "Front Panel.Title"=w535) -> (error out=w537:errorcluster)  [unwired: 1 out]
      }
      frame "CleansubPanel" {
        n214 = Unbundle By Name(w550) -> ("user event ref"=w549:T4)
        n215 = call "Remove UI without races.vi"("error in"=w551, "user event ref"=w549, "sub panel ref in"=w547) -> ("error out"=w548:errorcluster)  [unwired: 7 in, 1 out]
      }
      frame "ActivateNode" {
        n216 = Unbundle By Name(w559) -> ("user event ref"=w556:T4)
        n217 = call <vilib>:"Set Busy.vi"("error in (no error)"=w562) -> ("error out"=w554:errorcluster)  [unwired: 9 in, 1 out]
        n218 = call <vilib>:"IDtoNode.vi"("error in"=w554, "ID"=w563) -> ("error out"=w555:errorcluster, "invalid Id"=w558:bool, "node ref"=w557:T3)  [unwired: 7 in]
        n219 = case shown="False" w558 {
          tunnel: w557 -> [w570 _]
          tunnel: [w571 w574] -> w553
          tunnel: w555 -> [w568 w575]
          tunnel: w560 -> [w566 _]
          tunnel: w556 -> [w567 w572]
          tunnel: w552 -> [w564 w573]
          frame False {
            n220 = call "Remove UI without races.vi"("error in"=w568, "user event ref"=w567, "sub panel ref in"=w564) -> ("error out"=w569:errorcluster, "sub panel ref out"=w565:refnum<vi>)  [unwired: 7 in]
            n221 = call <vilib>:"LoadNodeUI.vi"("user event out"=w567, "error in"=w569, "sub panel ref in"=w565, "main queue"=w566, "node"=w570) -> ("error out"=w571:errorcluster)  [unwired: 6 in]
          }
          frame True {
            n222 = call "Remove UI without races.vi"("error in"=w575, "user event ref"=w572, "sub panel ref in"=w573) -> ("error out"=w574:errorcluster)  [unwired: 7 in, 1 out]
          }
        }
        n223 = call <vilib>:"Unset Busy.vi"("error in (no error)"=w553) -> ("error out"=w561:errorcluster)  [unwired: 10 in]
      }
      frame "Move" {
        n224 = Unflatten From String(type=T15 {"node ref"=refnum, "new parent"=refnum} ("Cluster"), binary string=w586, error in (no error)=w585) -> (value=w581:T15, error out=w580:errorcluster)  [unwired: 2 in, 1 out]
        n225 = Unbundle By Name(w581) -> ("node ref"=w577:T3, "new parent"=w576:T3)
        n226 = call <vilib>:"MoveNode.vi"("error in"=w580, "new parent"=w576, "node"=w577) -> ("error out"=w578:errorcluster)  [unwired: 8 in]
        n227 = call <vilib>:"Send Local Message.vi"("message queue in"=w583, "message name"="PopulateTree", "error in"=w578) -> ("error out"=w584:errorcluster)  [unwired: 10 in, 2 out]
      }
      frame "RefreshNodeView" {
        # "This user event is used by editor nodes to update their subpanels when data in the tree changes."
        n228 = Unbundle By Name(w589) -> ("user event ref"=w588:T4)
        n229 = Generate User Event(user event=w588, event data cluster=T8 {"command"="Refresh", "data"=""} ("event data"), error in=w591) -> (error out=w590:errorcluster)  [unwired: 1 in, 1 out]
      }
    }
  }
  n230 = while "User Interface Event Handler" {
    tunnel: w12 -> [w597]
    tunnel: w10 -> [w593]
    stop <- w596 stop-if-true
    n231 = event shown="[8] Menu Selection (User)" {
      selector: _ -> [_ _ _ _ _ _ _ _ _]
      dyn-events: _ -> [_ _ _ _ _ _ _ _ _]
      timeout: _ -> [_ _ _ _ _ _ _ _ _]
      tunnel: w597 -> [w605 w631 w673 w713 w720 w747 w751 w761 w766]
      tunnel: [_ _ _ TRUE _ _ _ _ _] -> w596
      tunnel: [w605 w623 w675 w709 w720 w744 w751 w759 w765] -> w595
      tunnel: [w600 w624 w674 w710 w716 w743 w748 w757 w763] -> w594
      tunnel: w593 -> [w604 w629 w672 w711 w719 w742 w750 w758 w764]
      event "View": Shortcut Menu Activation? {
        n232 = event-data() -> ("CtlRef"=w611:refnum<vi>, "Coords"=w610:T24, "MenuRef"=w607:refnum<k9>)  [unwired: 1 in]
        n233 = invoke class="Tree (strict)" method="Point To Row Column"(reference=w611, error in=w604, "Point"=w610) -> (error out=w603:errorcluster, "Tag"=w609:string)  [unwired: 5 in, 6 out]
        n234 = call <vilib>:"IDtoNode.vi"("error in"=w603, "ID"=w609) -> ("error out"=w601:errorcluster, "invalid Id"=w606:bool, "node ref"=w608:T3)  [unwired: 7 in]
        n235 = case shown="False" w606 {
          selector: w606 -> [_ w621]
          tunnel: w608 -> [w615 _]
          tunnel: w607 -> [w614 _]
          tunnel: [w613 _] -> w602
          tunnel: [w612 _] -> w599
          tunnel: [_ w621] -> w598
          frame False {
            n236 = in-place {
              in-place-border: w614 -> [w618]
              in-place-border: [w616] -> w613
              n237 = in-place-dvr #7(w615) -> (w620:refnum<class "NISE_CEF_Node.lvclass">, w617:errorcluster)
              n238 = call-dynamic "ShortcutMenu.vi"("error in"=w617, "menu ref in"=w618, "node in"=w620) -> ("error out"=w616:errorcluster, "node out"=w619:refnum<class "NISE_CEF_Node.lvclass">)  [unwired: 6 in, 1 out]
              n239 = in-place-dvr #7(w619) -> (w612:errorcluster)  [unwired: 1 out]
            }
          }
          frame True {
          }
        }
        n240 = Merge Errors(w599, w602, w601) -> (w600:errorcluster)
        n241 = event-data("Discard?"=w598) -> ()  [unwired: 1 in, 1 out]
      }
      event "View": Shortcut Menu Selection (User) {
        # "=nodeID"
        n242 = event-data() -> ("ItemPath"=w627:string, "CtlRef"=w634:refnum<vi>, "Coords"=w635:T24)  [unwired: 1 in]
        n243 = invoke class="Tree (strict)" method="Point To Row Column"(reference=w634, error in=w629, "Point"=w635) -> (error out=w628:errorcluster, "Tag"=w630:string)  [unwired: 5 in, 6 out]
        n244 = Match Pattern(string=w627, regular expression=":") -> (before substring=w633:string, after substring=w632:string)  [unwired: 1 in, 2 out]
        n245 = case shown="\"Add\"" w633 {
          tunnel: w632 -> [_ _ _ w664]
          tunnel: w631 -> [w642 w653 w659 w666]
          tunnel: w630 -> [w640 w647 w657 w665]
          tunnel: [w639 w651 w656 w662] -> w626
          tunnel: [w638 w650 w654 w660] -> w625
          tunnel: w628 -> [w637 w646 w655 w661]
          tunnel: w627 -> [_ w643 _ _]
          frame "Remove" {
            n246 = call <vilib>:"Send Local Message.vi"("message queue in"=w642, "message name"="RemoveNode" ("Message Name"), "message value"=w640, "error in"=w637) -> ("message queue out"=w639:T6, "error out"=w638:errorcluster)  [unwired: 9 in, 1 out]
          }
          frame Default {
            n247 = Bundle By Name(cluster=T13 {"node id"="", "RightClickPath"=""} ("input cluster"), "node id"=w647, "RightClickPath"=w643) -> (w648:T13)
            n248 = Flatten To String(anything=w648, error in (no error)=w646) -> (data string=w644:string, error out=w645:errorcluster)  [unwired: 2 in, 1 out]
            n249 = call <vilib>:"Send Local Message.vi"("message queue in"=w653, "message name"="HandleMenu" ("Message Name"), "message value"=w644, "error in"=w645) -> ("message queue out"=w651:T6, "error out"=w650:errorcluster)  [unwired: 9 in, 1 out]
          }
          frame "Duplicate" {
            n250 = call <vilib>:"Send Local Message.vi"("message queue in"=w659, "message name"="Duplicate" ("Message Name"), "message value"=w657, "error in"=w655) -> ("message queue out"=w656:T6, "error out"=w654:errorcluster)  [unwired: 9 in, 1 out]
          }
          frame "Add" {
            n251 = Bundle By Name(cluster=T14 {"node type"="", "to add to"=""} ("input cluster"), "node type"=w664, "to add to"=w665) -> (w667:T14)
            n252 = Flatten To String(anything=w667) -> (data string=w668:string)  [unwired: 3 in, 2 out]
            n253 = call <vilib>:"Send Local Message.vi"("message queue in"=w666, "message name"="AddNode" ("Message Name"), "message value"=w668, "error in"=w661) -> ("message queue out"=w662:T6, "error out"=w660:errorcluster)  [unwired: 9 in, 1 out]
          }
        }
        n254 = call <vilib>:"Send Local Message.vi"("message queue in"=w626, "message name"="RefreshNodeView", "error in"=w625) -> ("message queue out"=w623:T6, "error out"=w624:errorcluster)  [unwired: 10 in, 1 out]
      }
      event "View": Drop {
        n255 = event-data() -> ("CtlRef"=w671:refnum<vi>, "Coords"=w670:T24)  [unwired: 1 in]
        n256 = invoke class="Tree (strict)" method="Point To Row Column"(reference=w671, error in=w672, "Point"=w670) -> (reference out=w689:refnum<vi>, error out=w688:errorcluster, "Tag"=w685:string)  [unwired: 5 in, 5 out]
        n257 = call <vilib>:"ValidDragDrop.vi"("error in"=w688, "drag over"=w685, "tree ref in"=w689) -> ("error out"=w680:errorcluster, "accepted"=w683:bool, "drag"=w687:string, "tree ref out"=w690:refnum<vi>)  [unwired: 5 in]
        n258 = call <vilib>:"IDtoNode.vi"("error in"=w680, "ID"=w685) -> ("error out"=w681:errorcluster, "invalid Id"=w678:bool, "node ref"=w684:T3)  [unwired: 7 in]
        n259 = call <vilib>:"IDtoNode.vi"("error in"=w681, "ID"=w687) -> ("error out"=w679:errorcluster, "invalid Id"=w677:bool, "node ref"=w686:T3)  [unwired: 7 in]
        n260 = Compound Arithmetic op=AND(w683, invert w678, invert w677) -> (w682:bool)
        n261 = case shown="True" w682 {
          tunnel: w687 -> [_ w706]
          tunnel: w690 -> [_ w708]
          tunnel: [_ TRUE] -> w676
          tunnel: w685 -> [_ w704]
          tunnel: w673 -> [w692 w693]
          tunnel: [w692 w700] -> w675
          tunnel: [w691 w699] -> w674
          tunnel: w686 -> [_ w695]
          tunnel: w684 -> [_ w694]
          tunnel: w679 -> [w691 w696]
          frame False {
          }
          frame True {
            n262 = invoke class="Tree (strict)" method="Edit Tree Items.Move Item"(reference=w708, error in=w696, "tag"=w706, "New Parent"=w704) -> (error out=w697:errorcluster)  [unwired: 3 in, 6 out]
            n263 = Bundle By Name(cluster=T15 {"node ref"=refnum, "new parent"=refnum} ("Cluster"), "new parent"=w694, "node ref"=w695) -> (w703:T15)
            n264 = Flatten To String(anything=w703, error in (no error)=w697) -> (data string=w702:string, error out=w698:errorcluster)  [unwired: 2 in, 1 out]
            n265 = call <vilib>:"Send Local Message.vi"("message queue in"=w693, "message name"="Move", "message value"=w702, "error in"=w698) -> ("message queue out"=w700:T6, "error out"=w699:errorcluster)  [unwired: 9 in, 1 out]
          }
        }
        n266 = event-data("Accepted?"=w676) -> ()  [unwired: 1 in, 1 out]
      }
      event "Exit": Value Change {
        # "Exit the application                                           >> Stop this message generator loop    Cleaning errors if the other loop stop this one"
        n267 = event-data() -> ()  [unwired: 1 in, 1 out]
        n268 = call <vilib>:"Send Local Message.vi"("message queue in"=w713, "message name"="Close", "error in"=w711) -> ("message queue out"=w709:T6, "error out"=w714:errorcluster)  [unwired: 10 in, 1 out]
        n269 = call <vilib>:"Clear Errors.vi"("error in (no error)"=w714) -> ("error out"=w710:errorcluster)  [unwired: 6 in]
      }
      event "View": Drag Starting? {
        n270 = event-data() -> ("Data"=w726:T25, "CtlRef"=w728:refnum<vi>, "Coords"=w727:T24)  [unwired: 1 in]
        n271 = invoke class="Tree (strict)" method="Point To Row Column"(reference=w728, error in=w719, "Point"=w727) -> (error out=w718:errorcluster, "Tag"=w725:string)  [unwired: 5 in, 6 out]
        n272 = call <vilib>:"IDtoNode.vi"("error in"=w718, "ID"=w725) -> ("error out"=w717:errorcluster, "invalid Id"=w724:bool, "node ref"=w723:T3)  [unwired: 7 in]
        n273 = case shown="False" w724 {
          tunnel: w723 -> [w734 _]
          tunnel: [w731 TRUE ("Removable")] -> w721
          tunnel: w717 -> [w730 w740]
          tunnel: [w729 w740] -> w716
          frame False {
            n274 = in-place {
              in-place-border: [w737] -> w733
              in-place-border: w730 -> [w736]
              in-place-border: [w735] -> w729
              n275 = in-place-dvr #8(w734) -> (w739:refnum<class "NISE_CEF_Node.lvclass">)  [unwired: 1 out]
              n276 = call-dynamic "EditOptions.vi"("error in"=w736, "node in"=w739) -> ("error out"=w735:errorcluster, "edit options"=w737:T26, "node out"=w738:refnum<class "NISE_CEF_Node.lvclass">)  [unwired: 6 in, 1 out]
              n277 = in-place-dvr #8(w738) -> ()  [unwired: 2 out]
            }
            n278 = Unbundle By Name(w733) -> ("movable"=w732:bool)
            n279 = Not(x=w732) -> (.not. x?=w731:bool)
          }
          frame True {
          }
        }
        n280 = event-data("Data"=w726, "Drag Mode"=enum32{"copy or move", "copy only", "move only"}."move only", "Discard?"=w721) -> ()  [unwired: 1 in, 1 out]
      }
      event "View": Value Change {
        n281 = event-data() -> ("NewVal"=w745:string)  [unwired: 1 in]
        n282 = call <vilib>:"Send Local Message.vi"("message queue in"=w747, "message name"="ActivateNode" ("Message Name"), "message value"=w745, "error in"=w742) -> ("message queue out"=w744:T6, "error out"=w743:errorcluster)  [unwired: 9 in, 1 out]
      }
      event "View": event type 3.0.xa000003a {
        n283 = event-data() -> ("CtlRef"=w756:refnum<vi>, "Coords"=w753:T24)  [unwired: 1 in]
        n284 = invoke class="Tree (strict)" method="Point To Row Column"(reference=w756, error in=w750, "Point"=w753) -> (reference out=w755:refnum<vi>, error out=w749:errorcluster, "Tag"=w754:string)  [unwired: 5 in, 5 out]
        n285 = call <vilib>:"ValidDragDrop.vi"("error in"=w749, "drag over"=w754, "tree ref in"=w755) -> ("error out"=w748:errorcluster, "accepted"=w752:bool)  [unwired: 5 in, 2 out]
        n286 = event-data("Accepted?"=w752) -> ()  [unwired: 1 in, 1 out]
      }
      event Panel Close? {
        # "Intercepts the upper right close panel operation to allow a smooth shutdown as opposed to immediately killing the app."
        n287 = event-data() -> ()  [unwired: 1 in, 1 out]
        n288 = call <vilib>:"Send Local Message.vi"("message queue in"=w761, "message name"="Close?", "error in"=w758) -> ("message queue out"=w759:T6, "error out"=w757:errorcluster)  [unwired: 10 in, 1 out]
        n289 = event-data("Discard?"=TRUE) -> ()  [unwired: 1 in, 1 out]
      }
      event Menu Selection (User) {
        n290 = event-data() -> ("ItemPath"=w767:string)  [unwired: 1 in]
        n291 = case shown="\"_Tools:Script Include VI\"" w767 {
          tunnel: w766 -> [w769 w775 w780 w785 w790 w795 w804 w809 w814 w819 w824 w829 w835 w839]
          tunnel: [w769 w771 w776 w781 w786 w791 w801 w806 w811 w816 w821 w826 w832 w838] -> w765
          tunnel: w764 -> [w768 w773 w778 w783 w788 w793 w800 w807 w812 w817 w822 w827 w833 w837]
          tunnel: [w768 w772 w777 w782 w787 w792 w798 w805 w810 w815 w820 w825 w831 w836] -> w763
          frame Default {
            n292 = One Button Dialog(message="Unknown Menu Option") -> ()  [unwired: 1 in, 1 out]
          }
          frame "_File:_New" {
            n293 = call <vilib>:"Send Local Message.vi"("message queue in"=w775, "message name"="New?" ("Message Name"), "error in"=w773) -> ("message queue out"=w771:T6, "error out"=w772:errorcluster)  [unwired: 10 in, 1 out]
          }
          frame "_File:_Open" {
            n294 = call <vilib>:"Send Local Message.vi"("message queue in"=w780, "message name"="Open?" ("Message Name"), "error in"=w778) -> ("message queue out"=w776:T6, "error out"=w777:errorcluster)  [unwired: 10 in, 1 out]
          }
          frame "_File:_Save" {
            n295 = call <vilib>:"Send Local Message.vi"("message queue in"=w785, "message name"="Save" ("Message Name"), "error in"=w783) -> ("message queue out"=w781:T6, "error out"=w782:errorcluster)  [unwired: 10 in, 1 out]
          }
          frame "_File:Save As..." {
            n296 = call <vilib>:"Send Local Message.vi"("message queue in"=w790, "message name"="SaveAs" ("Message Name"), "error in"=w788) -> ("message queue out"=w786:T6, "error out"=w787:errorcluster)  [unwired: 10 in, 1 out]
          }
          frame "_File:_Exit" {
            n297 = call <vilib>:"Send Local Message.vi"("message queue in"=w795, "message name"="Close?" ("Message Name"), "error in"=w793) -> ("message queue out"=w791:T6, "error out"=w792:errorcluster)  [unwired: 10 in, 1 out]
          }
          frame "_Tools:Multiple Parameter Editor" {
            n298 = call <vilib>:"Send Local Message.vi"("message queue in"=w804, "message name"="CleansubPanel", "error in"=w800) -> ("message queue out"=w803:T6, "error out"=w799:errorcluster)  [unwired: 10 in, 1 out]
            n299 = call <vilib>:"Send Local Message.vi"("message queue in"=w803, "message name"="Custom View", "message value"="Multiple Parameter Editor" ("Message Name"), "error in"=w799) -> ("message queue out"=w801:T6, "error out"=w798:errorcluster)  [unwired: 9 in, 1 out]
          }
          frame "_Tools:Test" {
            n300 = call <vilib>:"Send Local Message.vi"("message queue in"=w809, "message name"="Test", "error in"=w807) -> ("message queue out"=w806:T6, "error out"=w805:errorcluster)  [unwired: 10 in, 1 out]
          }
          frame "_Tools:Deploy Tool" {
            n301 = call <vilib>:"Send Local Message.vi"("message queue in"=w814, "message name"="DeployTool", "error in"=w812) -> ("message queue out"=w811:T6, "error out"=w810:errorcluster)  [unwired: 10 in, 1 out]
          }
          frame "_Tools:Save Binary" {
            n302 = call <vilib>:"Send Local Message.vi"("message queue in"=w819, "message name"="Save Binary", "error in"=w817) -> ("message queue out"=w816:T6, "error out"=w815:errorcluster)  [unwired: 10 in, 1 out]
          }
          frame "_Tools:Script Include VI" {
            n303 = call <vilib>:"Send Local Message.vi"("message queue in"=w824, "message name"="Script Include VI", "error in"=w822) -> ("message queue out"=w821:T6, "error out"=w820:errorcluster)  [unwired: 10 in, 1 out]
          }
          frame "_Tools:Load Binary" {
            n304 = call <vilib>:"Send Local Message.vi"("message queue in"=w829, "message name"="Load Binary", "error in"=w827) -> ("message queue out"=w826:T6, "error out"=w825:errorcluster)  [unwired: 10 in, 1 out]
          }
          frame "_Tools:Refresh Plugins" {
            n305 = call <vilib>:"Send Local Message.vi"("message queue in"=w835, "message name"="FindPluginNodes", "message value"="Refresh", "error in"=w833) -> ("message queue out"=w832:T6, "error out"=w831:errorcluster)  [unwired: 9 in, 1 out]
          }
          frame "_Tools:Edit Plugin Search Paths" {
            n306 = call <vilib>:"Send Local Message.vi"("message queue in"=w839, "message name"="Edit Plugin Search Paths", "error in"=w837) -> ("message queue out"=w838:T6, "error out"=w836:errorcluster)  [unwired: 10 in, 1 out]
          }
        }
      }
    }
    n307 = call "send error message.vi"("error in"=w594, "message queue in"=w595) -> ()  [unwired: 9 in, 1 out]
  }
